vi "Comparacion de temperatura.vi"(2 "T2":dbl min=0.0 max=100.0 format="%#_4g", 3 "SP":u8 max=100) -> (0 "A":string caption="Actividad", 1 "C":string caption="Case")   [LabVIEW 2017]
doc: "Este VI realiza la comparacionentre la temperatura y el set point dado por el usuario dando a la salida una constante que equivale a uno de los casos de control ."
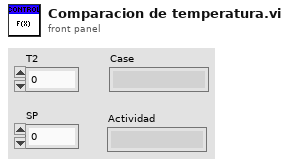
[diagram p1: front panel]
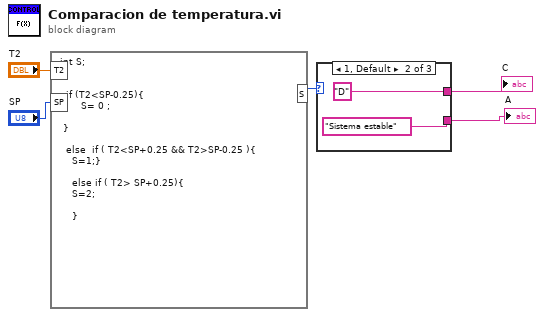
[diagram p0: block diagram]
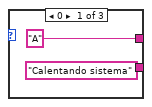
[diagram p2: hidden frame]
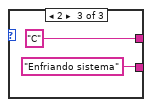
[diagram p3: hidden frame]
diagram:
  n1 = formula code="int S;\n\n\n  if (T2<SP-0.25){\n       S= 0 ; \n               \n }  \n\n  else  if ( T2<SP+0.25 && T2>SP-0.25 ){\n    S=1;}\n\n    else if ( T2> SP+0.25){\n    S=2;\n     \n    }"("T2"="T2", "SP"="SP") -> ("S"=w4:i32)
  n2 = case shown="1, Default" w4 {
    tunnel: ["A" "D" "C"] -> w5
    tunnel: ["Calentando sistema" "Sistema estable" "Enfriando sistema"] -> w1
    frame 0 {
    }
    frame 1, Default {
    }
    frame 2 {
    }
  }
  "C" <- w5
  "A" <- w1
